vi "log analysis_gps.vi"() -> ()   [LabVIEW 2019] (continued)
#DUALANTENNAHEADINGA,USB3,0,46.5,FINESTEERING,2107,282472.200,02000000,d426,15824;SOL_COMPUTED,L1_FLOAT,-1.000000000,54.732860565,-45.831329346,0.0,98.283119202,178.546401978,\"631T\",13,7,7,7,04,00,20,02*8ccffb99\n\tsystem status\tnormal 2 27.800000 0 0\trobot status\t337.454668\t28.997439\t11.768500\t0.229132\t0.985009\t-32.902606\t0.246000\t0.087000\n\t\n15:27:34.7\tlog_raw\tgps_raw\t#DUALANTENNAHEADINGA,USB3,0,46.5,FINESTEERING,2107,282472.700,02000000,d426,15824;SOL_COMPUTED,L1_FLOAT,-1.000000000,54.959995270,-45.596282959,0.0,98.333869934,179.821563721,\"631T\",13,7,7,7,04,00,20,02*00d3f37b\n\tsystem status\tnormal 2 27.800000 0 0\trobot status\t337.564510\t28.905721\t11.771200\t0.209692\t1.150870\t-32.233289\t0.308000\t-0.003000\n\t\n15:27:35.2\tlog_raw\tgps_raw\t#INSPVAXA,USB3,0,52.0,FINESTEERING,2107,282473.250,02000000,471d,15824;INS_ALIGNMENT_COMPLETE,INS_RTKFIXED,37.37038981275,126.72464739191,11.7746,22.3000,-0.1948,0.2277,0.0045,0.156747113,1.075368694,121.414050270,0.4373,0.2954,0.5425,0.1142,0.0935,0.0768,0.1366,0.1413,5.0978,0f000001,0*e88bca5a\n\tsystem status\tnormal 2 27.700000 0 0\trobot status\t337.686121\t28.806584\t11.774600\t0.156747\t1.075369\t-31.414050\t0.163000\t0.223000\n\t\n15:27:35.7\tlog_raw\tgps_raw\t#INSPVAXA,USB3,0,52.0,FINESTEERING,2107,282473.750,02000000,471d,15824;INS_ALIGNMENT_COMPLETE,INS_RTKFIXED,37.37038901794,126.72464863796,11.7783,22.3000,-0.1909,0.2328,0.0045,0.039175910,1.239409114,120.698239025,0.4373,0.2954,0.5425,0.1142,0.0935,0.0768,0.1366,0.1413,5.0978,0f000001,0*6f6aad10\n\tsystem status\tnormal 2 27.800000 0 0\trobot status\t337.796494\t28.718368\t11.778300\t0.039176\t1.239409\t-30.698239\t0.319000\t0.000000\n\t\n15:27:36.2\tlog_raw\tgps_raw\t#INSPVAXA,USB3,0,52.5,FINESTEERING,2107,282474.250,02000000,471d,15824;INS_ALIGNMENT_COMPLETE,INS_RTKFIXED,37.37038821663,126.72464993203,11.7822,22.3000,-0.1900,0.2213,-0.0032,0.050457416,1.361079347,119.957675424,0.4373,0.2953,0.5423,0.1143,0.0936,0.0767,0.1365,0.1412,5.0971,0f000001,0*04eefe7e\n\tsystem status\tnormal 2 27.800000 0 0\trobot status\t337.911121\t28.629430\t11.782200\t0.050457\t1.361079\t-29.957675\t0.355000\t-0.045000\n\t\n15:27:36.7\tlog_raw\tgps_raw\t#DUALANTENNAHEADINGA,USB3,0,52.5,FINESTEERING,2107,282474.700,02000000,d426,15824;SOL_COMPUTED,NARROW_FLOAT,-1.000000000,53.444328308,-36.252197266,0.0,99.495506287,180.000000000,\"631T\",13,7,7,7,04,00,20,03*a63b34b7\n\tsystem status\tnormal 2 27.800000 0 0\trobot status\t338.015790\t28.551056\t11.786100\t0.032591\t1.365886\t-29.248253\t0.330000\t-0.043000\n\t\n15:27:37.2\tlog_raw\tgps_raw\t\tsystem status\tnormal 2 27.800000 0 0\trobot status\t338.132602\t28.464845\t11.789800\t0.076114\t1.461863\t-28.564426\t0.425000\t-0.155000\n\t\n15:27:37.7\tlog_raw\tgps_raw\t#INSPVAXA,USB3,0,51.0,FINESTEERING,2107,282475.750,02000000,471d,15824;INS_ALIGNMENT_COMPLETE,INS_RTKFIXED,37.37038590363,126.72465390655,11.7950,22.3000,-0.1808,0.2394,-0.0047,0.109913426,1.377387594,117.860298903,0.4381,0.2954,0.5423,0.1145,0.0936,0.0767,0.1364,0.1410,5.0959,0f000001,0*7de89cb0\n\tsystem status\tnormal 2 27.800000 0 0\trobot status\t338.263177\t28.372709\t11.795000\t0.109913\t1.377388\t-27.860299\t0.307000\t-0.004000\n\t\n15:27:38.2\tlog_raw\tgps_raw\t#DUALANTENNAHEADINGA,USB3,0,51.5,FINESTEERING,2107,282476.200,02000000,d426,15824;SOL_COMPUTED,L1_FLOAT,-1.000000000,55.533638000,-0.375610352,0.0,117.860015869,180.000000000,\"631T\",14,7,7,7,04,00,20,02*d327ff6e\n\tsystem status\tnormal 2 27.800000 0 0\trobot status\t338.370911\t28.297956\t11.799000\t0.118267\t1.261755\t-27.251157\t0.371000\t-0.097000\n\t\n15:27:38.7\tlog_raw\tgps_raw\t#INSPVAXA,USB3,0,51.5,FINESTEERING,2107,282476.750,02000000,471d,15824;INS_ALIGNMENT_COMPLETE,INS_RTKFIXED,37.37038443010,126.72465662645,11.8037,22.3000,-0.1744,0.2321,0.0038,0.098053038,1.110033651,116.595542201,0.4382,0.2952,0.5423,0.1147,0.0936,0.0767,0.1363,0.1408,5.0950,0f000001,0*ea8caedb\n\tsystem status\tnormal 2 27.800000 0 0\trobot status\t338.504102\t28.209160\t11.803700\t0.098053\t1.110034\t-26.595542\t0.263000\t0.066000\n\t\n15:27:39.2\tlog_raw\tgps_raw\t#INSPVAXA,USB3,0,52.0,FINESTEERING,2107,282477.250,02000000,471d,15824;INS_ALIGNMENT_COMPLETE,INS_RTKFIXED,37.37038371373,126.72465798496,11.8086,22.3000,-0.1784,0.2376,0.0072,0.132722378,1.123390738,116.043560691,0.4382,0.2951,0.5421,0.1149,0.0937,0.0767,0.1362,0.1405,5.0949,0f000001,0*a21a9ce6\n\tsystem status\tnormal 2 27.800000 0 0\trobot status\t338.624436\t28.129649\t11.808600\t0.132722\t1.123391\t-26.043561\t0.236000\t0.120000\n\t\n15:27:39.7\tlog_raw\tgps_raw\t\tsystem status\tnormal 2 27.800000 0 0\trobot status\t338.734436\t28.057677\t11.812800\t0.158038\t0.982848\t-25.549618\t0.227000\t0.142000\n\t\n15:27:40.2\tlog_raw\tgps_raw\t#DUALANTENNAHEADINGA,USB3,0,47.5,FINESTEERING,2107,282478.200,02000000,d426,15824;SOL_COMPUTED,NARROW_FLOAT,-1.000000000,53.676605225,18.221975327,0.0,112.330833435,180.000000000,\"631T\",17,7,7,7,04,00,20,03*123ff075\n\tsystem status\tnormal 2 27.800000 0 0\trobot status\t338.855171\t27.980159\t11.816500\t0.150261\t1.168449\t-25.066939\t0.205000\t0.163000\n\t\n15:27:40.7\tlog_raw\tgps_raw\t#INSPVAXA,USB3,0,47.5,FINESTEERING,2107,282478.750,02000000,471d,15824;INS_ALIGNMENT_COMPLETE,INS_RTKFIXED,37.37038162641,126.72466209113,11.8198,22.3000,-0.1768,0.2383,-0.0098,0.146556317,1.371576994,114.526516784,0.4387,0.2951,0.5427,0.1151,0.0939,0.0768,0.1361,0.1403,5.0955,0f000001,0*9c50f9d9\n\tsystem status\tnormal 2 27.800000 0 0\trobot status\t338.988154\t27.897974\t11.819800\t0.146556\t1.371577\t-24.526517\t0.228000\t0.129000\n\t\n15:27:41.2\tlog_raw\tgps_raw\t#DUALANTENNAHEADINGA,USB3,0,50.0,FINESTEERING,2107,282479.200,02000000,d426,15824;SOL_COMPUTED,NARROW_FLOAT,-1.000000000,51.679660797,16.235267639,0.0,131.237731934,180.000000000,\"631T\",15,7,7,7,04,00,20,03*76498f9b\n\tsystem status\tnormal 2 27.900000 0 0\trobot status\t339.098405\t27.832776\t11.821900\t-0.028367\t1.309021\t-24.118833\t0.237000\t0.114000\n\t\n15:27:41.7\tlog_raw\tgps_raw\t#INSPVAXA,USB3,0,50.0,FINESTEERING,2107,282479.750,02000000,471d,15824;INS_ALIGNMENT_COMPLETE,INS_RTKFIXED,37.37038033615,126.72466486857,11.8253,22.3000,-0.1778,0.2630,-0.0031,-0.080326690,1.236523677,113.540262033,0.4414,0.2959,0.5454,0.1157,0.0941,0.0769,0.1359,0.1401,5.0966,0f000001,0*bc5588b9\n\tsystem status\tnormal 2 27.900000 0 0\trobot status\t339.234175\t27.754765\t11.825300\t-0.080327\t1.236524\t-23.540262\t0.233000\t0.109000\n\t\n15:27:42.2\tlog_raw\tgps_raw\t\tsystem status\tnormal 2 27.900000 0 0\trobot status\t339.345086\t27.692770\t11.827000\t-0.206343\t1.191786\t-23.092639\t0.254000\t0.074000\n\t\n15:27:42.7\tlog_raw\tgps_raw\t#INSPVAXA,USB3,0,51.0,FINESTEERING,2107,282480.750,02000000,471d,15824;INS_ALIGNMENT_COMPLETE,INS_RTKFIXED,37.37037910395,126.72466763539,11.8294,22.3000,-0.1682,0.2496,-0.0083,-0.123932791,1.123250163,112.586404178,0.4418,0.2960,0.5463,0.1157,0.0942,0.0770,0.1357,0.1398,5.0977,0f000001,0*a24ca24f\n\tsystem status\tnormal 2 27.900000 0 0\trobot status\t339.479256\t27.618000\t11.829400\t-0.123933\t1.123250\t-22.586404\t0.323000\t-0.027000\n\t\n15:27:43.2\tlog_raw\tgps_raw\t\tsystem status\tnormal 2 27.900000 0 0\trobot status\t339.593893\t27.557561\t11.831700\t-0.289570\t1.176785\t-22.187995\t0.299000\t0.006000\n\t\n15:27:43.7\tlog_raw\tgps_raw\t#INSPVAXA,USB3,0,49.5,FINESTEERING,2107,282481.750,02000000,471d,15824;INS_ALIGNMENT_COMPLETE,INS_RTKFIXED,37.37037789694,126.72467048931,11.8351,22.3000,-0.1461,0.2327,0.0043,-0.310804253,1.123961293,111.895191809,0.4415,0.2959,0.5463,0.1157,0.0942,0.0769,0.1355,0.1395,5.0988,0f000001,0*973dff57\n\tsystem status\tnormal 2 27.900000 0 0\trobot status\t339.732051\t27.484030\t11.835100\t-0.310804\t1.123961\t-21.895192\t0.346000\t-0.056000\n\t\n15:27:44.2\tlog_raw\tgps_raw\t#INSPVAXA,USB3,0,50.5,FINESTEERING,2107,282482.250,02000000,471d,15824;INS_ALIGNMENT_COMPLETE,INS_RTKFIXED,37.37037731116,126.72467190347,11.8384,22.3000,-0.1477,0.2523,-0.0105,-0.265666832,1.108878256,111.633485530,0.4404,0.2956,0.5456,0.1156,0.0941,0.0769,0.1353,0.1392,5.0999,0f000001,0*cd6558ee\n\tsystem status\tnormal 2 27.900000 0 0\trobot status\t339.857315\t27.419012\t11.838400\t-0.265667\t1.108878\t-21.633486\t0.243000\t0.085000\n\t\n15:27:44.7\tlog_raw\tgps_raw\t#INSPVAXA,USB3,0,50.5,FINESTEERING,2107,282482.750,02000000,471d,15824;INS_ALIGNMENT_COMPLETE,INS_RTKFIXED,37.37037674280,126.72467330399,11.8420,22.3000,-0.1430,0.2494,-0.0020,-0.174444219,1.137466494,111.346444953,0.4404,0.2956,0.5456,0.1156,0.0941,0.0769,0.1353,0.1392,5.0999,0f000001,0*2a49352f\n\tsystem status\tnormal 2 27.900000 0 0\trobot status\t339.981371\t27.355928\t11.842000\t-0.174444\t1.137466\t-21.346445\t0.276000\t0.036000\n\t\n15:27:45.2\tlog_raw\tgps_raw\t#INSPVAXA,USB3,0,50.0,FINESTEERING,2107,282483.250,02000000,471d,15824;INS_ALIGNMENT_COMPLETE,INS_RTKFIXED,37.37037616883,126.72467474324,11.8449,22.3000,-0.1483,0.2627,-0.0049,-0.159355428,1.028327028,111.093660255,0.4396,0.2956,0.5446,0.1155,0.0941,0.0768,0.1351,0.1389,5.1012,0f000001,0*e9226b16\n\tsystem status\tnormal 2 28.000000 0 0\trobot status\t340.108857\t27.292221\t11.844900\t-0.159355\t1.028327\t-21.093660\t0.334000\t-0.044000\n\t\n15:27:45.7\tlog_raw\tgps_raw\t#INSPVAXA,USB3,0,50.0,FINESTEERING,2107,282483.750,02000000,471d,15824;INS_ALIGNMENT_COMPLETE,INS_RTKFIXED,37.37037559924,126.72467616191,11.8460,22.3000,-0.1456,0.2485,-0.0071,-0.147252002,0.996738159,110.847183596,0.4396,0.2956,0.5446,0.1155,0.0941,0.0768,0.1351,0.1389,5.1012,0f000001,0*6063b49d\n\tsystem status\tnormal 2 28.000000 0 0\trobot status\t340.234521\t27.229000\t11.846000\t-0.147252\t0.996738\t-20.847184\t0.323000\t-0.029000\n\t\n15:27:46.2\tlog_raw\tgps_raw\t\tsystem status\tnormal 2 28.000000 0 0\trobot status\t340.347700\t27.173384\t11.848500\t-0.118940\t0.919299\t-20.556192\t0.292000\t0.033000\n\t\n15:27:46.7\tlog_raw\tgps_raw\t#INSPVAXA,USB3,0,51.5,FINESTEERING,2107,282484.750,02000000,471d,15824;INS_ALIGNMENT_COMPLETE,INS_RTKFIXED,37.37037448665,126.72467902626,11.8522,22.3000,-0.1407,0.2484,-0.0090,-0.064873099,1.145438573,110.168729835,0.4390,0.2955,0.5438,0.1153,0.0940,0.0767,0.1348,0.1386,5.1026,0f000001,0*a0636209\n\tsystem status\tnormal 2 27.900000 0 0\trobot status\t340.488240\t27.105510\t11.852200\t-0.064873\t1.145439\t-20.168730\t0.418000\t-0.152000\n\t\n15:27:47.2\tlog_raw\tgps_raw\t#INSPVAXA,USB3,0,51.0,FINESTEERING,2107,282485.250,02008000,471d,15824;INS_ALIGNMENT_COMPLETE,INS_RTKFIXED,37.37037393424,126.72468050363,11.8549,22.3000,-0.1324,0.2566,-0.0083,0.002695886,0.976355436,109.894464634,0.4390,0.2956,0.5434,0.1153,0.0939,0.0767,0.1346,0.1383,5.1041,0f000001,0*d70e669a\n\tsystem status\tnormal 2 27.900000 0 0\trobot status\t340.619103\t27.044195\t11.854900\t0.002696\t0.976355\t-19.894465\t0.328000\t-0.009000\n\t\n15:27:47.7\tlog_raw\tgps_raw\t#INSPVAXA,USB3,0,51.0,FINESTEERING,2107,282485.750,02008000,471d,15824;INS_ALIGNMENT_COMPLETE,INS_RTKFIXED,37.37037339561,126.72468193841,11.8561,22.3000,-0.1291,0.2465,-0.0040,0.117309078,0.863917654,109.567582429,0.4390,0.2956,0.5434,0.1153,0.0939,0.0767,0.1346,0.1383,5.1041,0f000001,0*167aa476\n\tsystem status\tnormal 2 27.900000 0 0\trobot status\t340.746194\t26.984411\t11.856100\t0.117309\t0.863918\t-19.567582\t0.358000\t-0.067000\n\t\n15:27:48.2\tlog_raw\tgps_raw\t#DUALANTENNAHEADINGA,USB3,0,52.0,FINESTEERING,2107,282486.200,02008000,d426,15824;SOL_COMPUTED,L1_FLOAT,-1.000000000,124.986564636,-52.100769043,0.0,360.000000000,180.000000000,\"631T\",12,6,6,6,04,00,20,02*25d98b4c\n\tsystem status\tnormal 2 27.900000 0 0\trobot status\t340.861761\t26.930390\t11.857200\t0.186163\t0.788623\t-19.301415\t0.403000\t-0.141000\n\t\n15:27:48.7\tlog_raw\tgps_raw\t#INSPVAXA,USB3,0,52.0,FINESTEERING,2107,282486.750,02008000,471d,15824;INS_ALIGNMENT_COMPLETE,INS_RTKFIXED,37.37037231578,126.72468487356,11.8580,22.3000,-0.1363,0.2539,-0.0079,0.065083536,0.658526684,108.961373177,0.4389,0.2956,0.5429,0.1152,0.0940,0.0767,0.1344,0.1380,5.1058,0f000001,0*795b201f\n\tsystem status\tnormal 2 27.900000 0 0\trobot status\t341.006184\t26.864555\t11.858000\t0.065084\t0.658527\t-18.961373\t0.271000\t0.041000\n\t\n15:27:49.2\tlog_raw\tgps_raw\t\tsystem status\tnormal 2 27.900000 0 0\trobot status\t341.122740\t26.810458\t11.859800\t0.109645\t0.579824\t-18.720730\t0.424000\t-0.184000\n\t\n15:27:49.7\tlog_raw\tgps_raw\t#INSPVAXA,USB3,0,53.0,FINESTEERING,2107,282487.750,02008000,471d,15824;INS_ALIGNMENT_COMPLETE,INS_RTKFIXED,37.37037124612,126.72468781330,11.8615,22.3000,-0.1351,0.2529,-0.0014,0.028036761,0.509941288,108.259170524,0.4390,0.2956,0.5427,0.1151,0.0939,0.0767,0.1342,0.1378,5.1072,0f000001,0*7116cc62\n\tsystem status\tnormal 2 27.900000 0 0\trobot status\t341.266582\t26.745829\t11.861500\t0.028037\t0.509941\t-18.259171\t0.398000\t-0.147000\n\t\n15:27:50.2\tlog_raw\tgps_raw\t\tsystem status\tnormal 2 27.900000 0 0\trobot status\t341.382407\t26.694008\t11.863500\t0.059660\t0.738081\t-17.950165\t0.237000\t0.109000\n\t\n15:27:50.7\tlog_raw\tgps_raw\t#INSPVAXA,USB3,0,50.5,FINESTEERING,2107,282488.750,02008000,471d,15824;INS_ALIGNMENT_COMPLETE,INS_RTKFIXED,37.37037023523,126.72469074006,11.8656,22.3000,-0.1204,0.2670,0.0002,0.044873893,0.831014389,107.580535120,0.4389,0.2956,0.5425,0.1150,0.0937,0.0767,0.1339,0.1375,5.1082,0f000001,0*4cab4b69\n\tsystem status\tnormal 2 27.900000 0 0\trobot status\t341.525829\t26.633625\t11.865600\t0.044874\t0.831014\t-17.580535\t0.245000\t0.092000\n\t\n15:27:51.2\tlog_raw\tgps_raw\t#INSPVAXA,USB3,0,51.0,FINESTEERING,2107,282489.250,02000000,471d,15824;INS_ALIGNMENT_COMPLETE,INS_RTKFIXED,37.37036974630,126.72469219938,11.8668,22.3000,-0.1082,0.2562,0.0055,0.037042210,0.796968035,107.199262674,0.4392,0.2956,0.5428,0.1149,0.0936,0.0767,0.1337,0.1373,5.1092,0f000001,0*9fc09916\n\tsystem status\tnormal 2 27.900000 0 0\trobot status\t341.655094\t26.579356\t11.866800\t0.037042\t0.796968\t-17.199263\t0.281000\t0.033000\n\t\n15:27:51.7\tlog_raw\tgps_raw\t\tsystem status\tnormal 2 27.900000 0 0\trobot status\t341.772406\t26.530600\t11.867400\t-0.037262\t1.019759\t-16.874243\t0.281000\t0.031000\n\t\n15:27:52.2\tlog_raw\tgps_raw\t#INSPVAXA,USB3,0,52.0,FINESTEERING,2107,282490.250,02000000,471d,15824;INS_ALIGNMENT_COMPLETE,INS_RTKFIXED,37.37036877450,126.72469515177,11.8697,22.3000,-0.1086,0.2580,0.0081,-0.074758775,1.106093430,106.454761549,0.4393,0.2955,0.5430,0.1148,0.0934,0.0768,0.1335,0.1371,5.1102,0f000001,0*37127645\n\tsystem status\tnormal 2 27.900000 0 0\trobot status\t341.916611\t26.471491\t11.869700\t-0.074759\t1.106093\t-16.454762\t0.203000\t0.151000\n\t\n15:27:52.7\tlog_raw\tgps_raw\t#INSPVAXA,USB3,0,52.0,FINESTEERING,2107,282490.750,02000000,471d,15824;INS_ALIGNMENT_COMPLETE,INS_RTKFIXED,37.37036829389,126.72469663971,11.8737,22.3000,-0.1049,0.2625,0.0062,-0.116881471,1.024892331,106.058307514,0.4393,0.2955,0.5430,0.1148,0.0934,0.0768,0.1335,0.1371,5.1102,0f000001,0*7841381f\n\tsystem status\tnormal 2 27.900000 0 0\trobot status\t342.048411\t26.418145\t11.873700\t-0.116881\t1.024892\t-16.058308\t0.269000\t0.064000\n\t\n15:27:53.2\tlog_raw\tgps_raw\t#INSPVAXA,USB3,0,51.5,FINESTEERING,2107,282491.250,02000000,471d,15824;INS_ALIGNMENT_COMPLETE,INS_RTKFIXED,37.37036783071,126.72469814477,11.8773,22.3000,-0.1005,0.2703,0.0019,-0.302758145,0.967035823,105.571562776,0.4390,0.2953,0.5427,0.1146,0.0933,0.0767,0.1334,0.1370,5.1117,0f000001,0*df8a40e1\n\tsystem status\tnormal 2 28.000000 0 0\trobot status\t342.181726\t26.366734\t11.877300\t-0.302758\t0.967036\t-15.571563\t0.275000\t0.058000\n\t\n15:27:53.7\tlog_raw\tgps_raw\t\tsystem status\tnormal 2 27.900000 0 0\trobot status\t342.301044\t26.320984\t11.881500\t-0.457558\t0.959747\t-15.154789\t0.307000\t0.003000\n\t\n15:27:54.2\tlog_raw\tgps_raw\t#INSPVAXA,USB3,0,53.0,FINESTEERING,2107,282492.250,02000000,471d,15824;INS_ALIGNMENT_COMPLETE,INS_RTKFIXED,37.37036690492,126.72470114805,11.8868,22.3000,-0.1128,0.2686,-0.0005,-0.341749532,1.011987346,104.657671438,0.4386,0.2951,0.5424,0.1145,0.0933,0.0767,0.1332,0.1368,5.1133,0f000001,0*36e30592\n\tsystem status\tnormal 2 27.900000 0 0\trobot status\t342.447752\t26.263974\t11.886800\t-0.341750\t1.011987\t-14.657671\t0.395000\t-0.113000\n\t\n15:27:54.7\tlog_raw\tgps_raw\t#INSPVAXA,USB3,0,53.0,FINESTEERING,2107,282492.750,02000000,471d,15824;INS_ALIGNMENT_COMPLETE,INS_RTKFIXED,37.37036645131,126.72470265161,11.8901,22.3000,-0.1035,0.2695,-0.0047,-0.206753293,0.813426880,104.258109250,0.4386,0.2951,0.5424,0.1145,0.0933,0.0767,0.1332,0.1368,5.1133,0f000001,0*577226f1\n\tsystem status\tnormal 2 27.900000 0 0\trobot status\t342.580935\t26.213625\t11.890100\t-0.206753\t0.813427\t-14.258109\t0.242000\t0.099000\n\t\n15:27:55.2\tlog_raw\tgps_raw\t#INSPVAXA,USB3,0,50.0,FINESTEERING,2107,282493.250,02000000,471d,15824;INS_ALIGNMENT_COMPLETE,INS_RTKFIXED,37.37036601456,126.72470416352,11.8919,22.3000,-0.1012,0.2672,-0.0093,-0.224228213,0.685864648,103.742995644,0.4383,0.2950,0.5422,0.1144,0.0932,0.0767,0.1331,0.1366,5.1149,0f000001,0*31397ff1\n\tsystem status\tnormal 2 27.800000 0 0\trobot status\t342.714857\t26.165147\t11.891900\t-0.224228\t0.685865\t-13.742996\t0.219000\t0.126000\n\t\n15:27:55.7\tlog_raw\tgps_raw\t#INSPVAXA,USB3,0,50.0,FINESTEERING,2107,282493.750,02000000,471d,15824;INS_ALIGNMENT_COMPLETE,INS_RTKFIXED,37.37036559899,126.72470566002,11.8945,22.3000,-0.1067,0.2704,-0.0029,-0.332770610,0.803747172,103.266979310,0.4383,0.2950,0.5422,0.1144,0.0932,0.0767,0.1331,0.1366,5.1149,0f000001,0*9ccbb3e3\n\tsystem status\tnormal 2 27.800000 0 0\trobot status\t342.847415\t26.119020\t11.894500\t-0.332771\t0.803747\t-13.266979\t0.254000\t0.083000\n\t\n15:27:56.2\tlog_raw\tgps_raw\t#INSPVAXA,USB3,0,54.0,FINESTEERING,2107,282494.250,02000000,471d,15824;INS_ALIGNMENT_COMPLETE,INS_RTKFIXED,37.37036518833,126.72470716061,11.8982,22.3000,-0.0992,0.2825,-0.0009,-0.390155029,0.844314939,102.750620694,0.4383,0.2950,0.5423,0.1144,0.0933,0.0767,0.1329,0.1365,5.1164,0f000001,0*37164162\n\tsystem status\tnormal 2 27.900000 0 0\trobot status\t342.980335\t26.073438\t11.898200\t-0.390155\t0.844315\t-12.750621\t0.238000\t0.095000\n\t\n15:27:56.7\tlog_raw\tgps_raw\t#INSPVAXA,USB3,0,54.0,FINESTEERING,2107,282494.750,02000000,471d,15824;INS_ALIGNMENT_COMPLETE,INS_RTKFIXED,37.37036477713,126.72470868073,11.9009,22.3000,-0.0879,0.2706,0.0036,-0.341565952,0.784824904,102.134248180,0.4383,0.2950,0.5423,0.1144,0.0933,0.0767,0.1329,0.1365,5.1164,0f000001,0*6a9baff3\n\tsystem status\tnormal 2 27.800000 0 0\trobot status\t343.114985\t26.027795\t11.900900\t-0.341566\t0.784825\t-12.134248\t0.294000\t0.017000\n\t\n15:27:57.2\tlog_raw\tgps_raw\t\tsystem status\tnormal 2 27.800000 0 0\trobot status\t343.237786\t25.988898\t11.902700\t-0.374669\t0.912618\t-11.541175\t0.272000\t0.062000\n\t\n15:27:57.7\tlog_raw\tgps_raw\t#INSPVAXA,USB3,0,52.0,FINESTEERING,2107,282495.750,02000000,471d,15824;INS_ALIGNMENT_COMPLETE,INS_RTKFIXED,37.37036401120,126.72471176105,11.9046,22.3000,-0.0834,0.2786,-0.0076,-0.308157155,0.761064852,100.941117040,0.4380,0.2949,0.5422,0.1143,0.0933,0.0767,0.1328,0.1363,5.1178,0f000001,0*054ad5c7\n\tsystem status\tnormal 2 27.800000 0 0\trobot status\t343.387834\t25.942777\t11.904600\t-0.308157\t0.761065\t-10.941117\t0.298000\t0.027000\n\t\n15:27:58.2\tlog_raw\tgps_raw\t#INSPVAXA,USB3,0,50.5,FINESTEERING,2107,282496.250,02000000,471d,15824;INS_ALIGNMENT_COMPLETE,INS_RTKFIXED,37.37036364901,126.72471328274,11.9089,22.3000,-0.0739,0.2539,-0.0014,-0.343894984,0.754370105,100.232900120,0.4379,0.2949,0.5421,0.1143,0.0933,0.0767,0.1327,0.1362,5.1190,0f000001,0*8784bafb\n\tsystem status\tnormal 2 27.800000 0 0\trobot status\t343.522623\t25.902574\t11.908900\t-0.343895\t0.754370\t-10.232900\t0.196000\t0.177000\n\t\n15:27:58.7\tlog_raw\tgps_raw\t#INSPVAXA,USB3,0,50.5,FINESTEERING,2107,282496.750,02000000,471d,15824;INS_ALIGNMENT_COMPLETE,INS_RTKFIXED,37.37036328787,126.72471481476,11.9136,22.3000,-0.0700,0.2693,-0.0009,-0.270371003,0.729660939,99.468887752,0.4379,0.2949,0.5421,0.1143,0.0933,0.0767,0.1327,0.1362,5.1190,0f000001,0*224a36a2\n\tsystem status\tnormal 2 27.800000 0 0\trobot status\t343.658327\t25.862488\t11.913600\t-0.270371\t0.729661\t-9.468888\t0.272000\t0.081000\n\t\n15:27:59.2\tlog_raw\tgps_raw\t#INSPVAXA,USB3,0,52.0,FINESTEERING,2107,282497.250,02000000,471d,15824;INS_ALIGNMENT_COMPLETE,INS_RTKFIXED,37.37036295953,126.72471635660,11.9170,22.3000,-0.0692,0.2638,0.0039,-0.487791758,0.697577068,98.688104249,0.4380,0.2950,0.5422,0.1144,0.0934,0.0767,0.1326,0.1361,5.1201,0f000001,0*5983bd1e\n\tsystem status\tnormal 2 27.800000 0 0\trobot status\t343.794901\t25.826042\t11.917000\t-0.487792\t0.697577\t-8.688104\t0.232000\t0.118000\n\t\n15:27:59.7\tlog_raw\tgps_raw\t#INSPVAXA,USB3,0,52.0,FINESTEERING,2107,282497.750,02000000,471d,15824;INS_ALIGNMENT_COMPLETE,INS_RTKFIXED,37.37036264142,126.72471787968,11.9197,22.3000,-0.0695,0.2760,-0.0054,-0.578412192,0.764831938,97.837503717,0.4380,0.2950,0.5422,0.1144,0.0934,0.0767,0.1326,0.1361,5.1201,0f000001,0*bf0827fb\n\tsystem status\tnormal 2 27.700000 0 0\trobot status\t343.929812\t25.790731\t11.919700\t-0.578412\t0.764832\t-7.837504\t0.312000\t0.003000\n\t\n15:28:00.2\tlog_raw\tgps_raw\t#INSPVAXA,USB3,0,50.5,FINESTEERING,2107,282498.250,02000000,471d,15824;INS_ALIGNMENT_COMPLETE,INS_RTKFIXED,37.37036233909,126.72471942444,11.9220,22.3000,-0.0554,0.2842,0.0042,-0.538460345,0.850776558,96.860804388,0.4376,0.2949,0.5421,0.1145,0.0934,0.0767,0.1325,0.1359,5.1211,0f000001,0*e69b7700\n\tsystem status\tnormal 2 27.700000 0 0\trobot status\t344.066645\t25.757171\t11.922000\t-0.538460\t0.850777\t-6.860804\t0.217000\t0.149000\n\t\n15:28:00.7\tlog_raw\tgps_raw\t#INSPVAXA,USB3,0,50.5,FINESTEERING,2107,282498.750,02000000,471d,15824;INS_ALIGNMENT_COMPLETE,INS_RTKFIXED,37.37036207253,126.72472096393,11.9246,22.3000,-0.0513,0.2714,0.0039,-0.548055416,0.760878793,95.595246784,0.4376,0.2949,0.5421,0.1145,0.0934,0.0767,0.1325,0.1359,5.1211,0f000001,0*75d334ae\n\tsystem status\tnormal 2 27.700000 0 0\trobot status\t344.203010\t25.727581\t11.924600\t-0.548055\t0.760879\t-5.595247\t0.291000\t0.035000\n\t\n15:28:01.2\tlog_raw\tgps_raw\t#INSPVAXA,USB3,0,51.0,FINESTEERING,2107,282499.250,02000000,471d,15824;INS_ALIGNMENT_COMPLETE,INS_RTKFIXED,37.37036182665,126.72472251722,11.9274,22.3000,-0.0518,0.2707,0.0042,-0.612176508,0.765223252,94.525809257,0.4377,0.2950,0.5421,0.1146,0.0936,0.0767,0.1324,0.1357,5.1220,0f000001,0*ec8d0c0f\n\tsystem status\tnormal 2 27.600000 0 0\trobot status\t344.340598\t25.700287\t11.927400\t-0.612177\t0.765223\t-4.525809\t0.294000\t0.038000\n\t\n15:28:01.7\tlog_raw\tgps_raw\t#INSPVAXA,USB3,0,51.0,FINESTEERING,2107,282499.750,02000000,471d,15824;INS_ALIGNMENT_COMPLETE,INS_RTKFIXED,37.37036160600,126.72472408768,11.9291,22.3000,-0.0494,0.2821,-0.0083,-0.781502529,0.706412197,93.339152024,0.4377,0.2950,0.5421,0.1146,0.0936,0.0767,0.1324,0.1357,5.1220,0f000001,0*d9b69855\n\tsystem status\tnormal 2 27.700000 0 0\trobot status\t344.479707\t25.675792\t11.929100\t-0.781503\t0.706412\t-3.339152\t0.303000\t0.039000\n\t\n15:28:02.2\tlog_raw\tgps_raw\t#INSPVAXA,USB3,0,53.0,FINESTEERING,2107,282500.250,02000000,471d,15824;INS_ALIGNMENT_COMPLETE,INS_RTKFIXED,37.37036138755,126.72472565119,11.9317,22.3000,-0.0342,0.2702,0.0095,-0.593682831,0.623847561,91.416153722,0.4373,0.2951,0.5419,0.1148,0.0938,0.0767,0.1322,0.1355,5.1229,0f000001,0*07814bab\n\tsystem status\tnormal 2 27.400000 0 0\trobot status\t344.618200\t25.651542\t11.931700\t-0.593683\t0.623848\t-1.416154\t0.290000\t0.144000\n\t\n15:28:02.7\tlog_raw\tgps_raw\t#INSPVAXA,USB3,0,53.0,FINESTEERING,2107,282500.750,02000000,471d,15824;INS_ALIGNMENT_COMPLETE,INS_RTKFIXED,37.37036130198,126.72472720567,11.9351,22.3000,0.0292,0.2886,0.0019,-0.781993907,0.527535072,86.351201750,0.4373,0.2951,0.5419,0.1148,0.0938,0.0767,0.1322,0.1355,5.1229,0f000001,0*6a6ac25a\n\tsystem status\tnormal 2 27.200000 0 0\trobot status\t344.755893\t25.642039\t11.935100\t-0.781994\t0.527535\t3.648798\t0.283000\t0.183000\n\t\n15:28:03.2\tlog_raw\tgps_raw\t#INSPVAXA,USB3,0,50.5,FINESTEERING,2107,282501.250,02000000,471d,15824;INS_ALIGNMENT_COMPLETE,INS_RTKFIXED,37.37036131745,126.72472879768,11.9390,22.3000,0.0369,0.2857,-0.0120,-0.997390809,0.433664742,81.039166738,0.4370,0.2954,0.5418,0.1155,0.0947,0.0767,0.1321,0.1353,5.1226,0f000001,0*2c9768ec\n\tsystem status\tnormal 2 27.100000 4 0\trobot status\t344.896911\t25.643751\t11.939000\t-0.997391\t0.433665\t8.960833\t0.311000\t0.166000\n\t\n15:28:03.7\tlog_raw\tgps_raw\t#INSPVAXA,USB3,0,50.5,FINESTEERING,2107,282501.750,02000000,471d,15824;INS_ALIGNMENT_COMPLETE,INS_RTKFIXED,37.37036141879,126.72473040754,11.9428,22.3000,0.0024,0.2788,-0.0052,-1.183204075,0.224327122,76.081887809,0.4370,0.2954,0.5418,0.1155,0.0947,0.0767,0.1321,0.1353,5.1226,0f000001,0*e82bc0a6\n\tsystem status\tnormal 2 27.300000 4 0\trobot status\t345.039510\t25.654992\t11.942800\t-1.183204\t0.224327\t13.918112\t0.325000\t0.168000\n\t\n15:28:04.2\tlog_raw\tgps_raw\t#INSPVAXA,USB3,0,52.5,FINESTEERING,2107,282502.250,02000000,471d,15824;INS_ALIGNMENT_COMPLETE,INS_RTKFIXED,37.37036164481,126.72473194519,11.9462,22.3000,0.0415,0.2803,0.0079,-1.160166771,-0.046948160,70.699699998,0.4369,0.2959,0.5417,0.1169,0.0967,0.0767,0.1320,0.1349,5.1194,0f000001,0*06dae310\n\tsystem status\tnormal 2 27.200000 4 0\trobot status\t345.175712\t25.680071\t11.946200\t-1.160167\t-0.046948\t19.300300\t0.313000\t0.172000\n\t\n15:28:04.7\tlog_raw\tgps_raw\t#INSPVAXA,USB3,0,52.5,FINESTEERING,2107,282502.750,02000000,471d,15824;INS_ALIGNMENT_COMPLETE,INS_RTKFIXED,37.37036200144,126.72473343849,11.9497,22.3000,0.0229,0.2449,0.0184,-1.242261291,-0.215624383,65.570089717,0.4369,0.2959,0.5417,0.1169,0.0967,0.0767,0.1320,0.1349,5.1194,0f000001,0*37a9ba1d\n\tsystem status\tnormal 2 27.100000 4 0\trobot status\t345.307986\t25.719646\t11.949700\t-1.242261\t-0.215624\t24.429910\t0.318000\t0.242000\n\t\n15:28:05.2\tlog_raw\tgps_raw\t#INSPVAXA,USB3,0,50.0,FINESTEERING,2107,282503.250,02000000,471d,15824;INS_ALIGNMENT_COMPLETE,INS_RTKFIXED,37.37036244144,126.72473485715,11.9546,22.3000,0.1159,0.2427,0.0087,-1.370274877,-0.522424319,60.146587364,0.4368,0.2966,0.5416,0.1192,0.0988,0.0767,0.1318,0.1345,5.1111,0f000001,0*9f9b3eba\n\tsystem status\tnormal 2 27.200000 4 0\trobot status\t345.433649\t25.768474\t11.954600\t-1.370275\t-0.522424\t29.853413\t0.306000\t0.172000\n\t\n15:28:05.7\tlog_raw\tgps_raw\t#INSPVAXA,USB3,0,50.0,FINESTEERING,2107,282503.750,02000000,471d,15824;INS_ALIGNMENT_COMPLETE,INS_RTKFIXED,37.37036302784,126.72473625079,11.9579,22.3000,0.1573,0.2456,0.0068,-1.326431987,-0.638529875,54.895159113,0.4368,0.2966,0.5416,0.1192,0.0988,0.0767,0.1318,0.1345,5.1111,0f000001,0*c3a1e695\n\tsystem status\tnormal 2 27.300000 4 0\trobot status\t345.557095\t25.833550\t11.957900\t-1.326432\t-0.638530\t35.104841\t0.298000\t0.165000\n\t\n15:28:06.2\tlog_raw\tgps_raw\t#INSPVAXA,USB3,0,51.0,FINESTEERING,2107,282504.250,02000000,471d,15824;INS_ALIGNMENT_COMPLETE,INS_RTKFIXED,37.37036369327,126.72473758611,11.9611,22.3000,0.1628,0.2237,0.0021,-1.236535008,-0.784458797,49.797084734,0.4377,0.2981,0.5419,0.1224,0.1023,0.0767,0.1314,0.1337,5.1002,0f000001,0*ce2dc0c6\n\tsystem status\tnormal 2 27.200000 4 0\trobot status\t345.675376\t25.907398\t11.961100\t-1.236535\t-0.784459\t40.202915\t0.310000\t0.175000\n\t\n15:28:06.7\tlog_raw\tgps_raw\t#INSPVAXA,USB3,0,51.0,FINESTEERING,2107,282504.750,02000000,471d,15824;INS_ALIGNMENT_COMPLETE,INS_RTKFIXED,37.37036443928,126.72473881419,11.9655,22.3000,0.1771,0.2224,-0.0093,-1.091153284,-0.604631231,44.754867869,0.4377,0.2981,0.5419,0.1224,0.1023,0.0767,0.1314,0.1337,5.1002,0f000001,0*68fd2785\n\tsystem status\tnormal 2 27.200000 4 0\trobot status\t345.784157\t25.990189\t11.965500\t-1.091153\t-0.604631\t45.245132\t0.332000\t0.139000\n\t\n15:28:07.2\tlog_raw\tgps_raw\t#INSPVAXA,USB3,0,51.0,FINESTEERING,2107,282505.250,02000000,471d,15824;INS_ALIGNMENT_COMPLETE,INS_RTKFIXED,37.37036527959,126.72473995022,11.9707,22.3000,0.1963,0.1952,-0.0121,-1.138350697,-0.474117376,39.571733238,0.4394,0.3003,0.5422,0.1267,0.1058,0.0767,0.1307,0.1325,5.0879,0f000001,0*6827ef91\n\tsystem status\tnormal 2 27.100000 4 0\trobot status\t345.884785\t26.083446\t11.970700\t-1.138351\t-0.474117\t50.428267\t0.287000\t0.194000\n\t\n15:28:07.7\tlog_raw\tgps_raw\t#INSPVAXA,USB3,0,51.0,FINESTEERING,2107,282505.750,02000000,471d,15824;INS_ALIGNMENT_COMPLETE,INS_RTKFIXED,37.37036623616,126.72474098646,11.9763,22.3000,0.2120,0.1861,0.0048,-1.165263195,-0.362025094,34.418588384,0.4394,0.3003,0.5422,0.1267,0.1058,0.0767,0.1307,0.1325,5.0879,0f000001,0*40d9afbc\n\tsystem status\tnormal 2 27.200000 4 0\trobot status\t345.976573\t26.189607\t11.976300\t-1.165263\t-0.362025\t55.581412\t0.326000\t0.171000\n\t\n15:28:08.2\tlog_raw\tgps_raw\t#INSPVAXA,USB3,0,51.5,FINESTEERING,2107,282506.250,02000000,471d,15824;INS_ALIGNMENT_COMPLETE,INS_RTKFIXED,37.37036720685,126.72474192456,11.9800,22.3000,0.2212,0.1614,0.0108,-1.132985321,-0.180413000,28.958926810,0.4417,0.3033,0.5424,0.1317,0.1100,0.0768,0.1296,0.1309,5.0779,0f000001,0*2e0d677d\n\tsystem status\tnormal 2 27.200000 4 0\trobot status\t346.059669\t26.297335\t11.980000\t-1.132985\t-0.180413\t61.041073\t0.302000\t0.181000\n\t\n15:28:08.7\tlog_raw\tgps_raw\t#INSPVAXA,USB3,0,51.5,FINESTEERING,2107,282506.750,02000000,471d,15824;INS_ALIGNMENT_COMPLETE,INS_RTKFIXED,37.37036827241,126.72474279747,11.9819,22.3000,0.2642,0.1305,0.0010,-1.072910910,-0.236865707,23.702771649,0.4417,0.3033,0.5424,0.1317,0.1100,0.0768,0.1296,0.1309,5.0779,0f000001,0*c0c775a0\n\tsystem status\tnormal 2 27.100000 4 0\trobot status\t346.136989\t26.415593\t11.981900\t-1.072911\t-0.236866\t66.297228\t0.282000\t0.216000\n\t\n15:28:09.2\tlog_raw\tgps_raw\t#INSPVAXA,USB3,0,51.0,FINESTEERING,2107,282507.250,02000000,471d,15824;INS_ALIGNMENT_COMPLETE,INS_RTKFIXED,37.37036943623,126.72474351475,11.9844,22.3000,0.2890,0.1143,0.0134,-1.116078326,-0.545577808,18.460028821,0.4448,0.3070,0.5424,0.1371,0.1144,0.0767,0.1279,0.1286,5.0714,0f000001,0*f2488cfe\n\tsystem status\tnormal 2 27.000000 4 0\trobot status\t346.200525\t26.544756\t11.984400\t-1.116078\t-0.545578\t71.539971\t0.318000\t0.148000\n\t\n15:28:09.7\tlog_raw\tgps_raw\t\tsystem status\texception 2 27.700000 4 160\trobot status\t346.243737\t26.612990\t11.986800\t-0.886764\t-0.668691\t73.434057\t0.120000\t-0.067000\n\t\n15:28:10.2\tlog_raw\tgps_raw\t#INSPVAXA,USB3,0,49.5,FINESTEERING,2107,282508.250,02000000,471d,15824;INS_ALIGNMENT_COMPLETE,INS_RTKFIXED,37.37036997810,126.72474418441,11.9888,22.3000,-0.0010,0.0343,0.0051,-0.948239100,-0.592787875,16.930139244,0.4486,0.3110,0.5423,0.1420,0.1207,0.0767,0.1255,0.1258,5.0683,0f000001,0*51dd059e\n\tsystem status\texception 2 28.000000 0 160\trobot status\t346.259842\t26.604893\t11.988800\t-0.948239\t-0.592788\t73.069861\t0.103000\t0.156000\n\t\n15:28:10.7\tlog_raw\tgps_raw\t#INSPVAXA,USB3,0,49.5,FINESTEERING,2107,282508.750,02000000,471d,15824;INS_ALIGNMENT_COMPLETE,INS_RTKFIXED,37.37036994386,126.72474436952,11.9909,22.3000,0.0056,0.0342,0.0053,-0.946500303,-0.592283051,16.912290627,0.4486,0.3110,0.5423,0.1420,0.1207,0.0767,0.1255,0.1258,5.0683,0f000001,0*09452605\n\tsystem status\texception 2 28.000000 0 160\trobot status\t346.276239\t26.601092\t11.990900\t-0.946500\t-0.592283\t73.087709\t0.103000\t0.156000\n\t\n15:28:11.2\tlog_raw\tgps_raw\t#INSPVAXA,USB3,0,51.0,FINESTEERING,2107,282509.250,02000000,471d,15824;INS_ALIGNMENT_COMPLETE,INS_RTKFIXED,37.37036993090,126.72474452786,11.9926,22.3000,0.0102,0.0361,0.0058,-0.944896447,-0.590729782,16.915447262,0.4529,0.3176,0.5421,0.1446,0.1223,0.0767,0.1224,0.1224,5.0667,0f000001,0*6e2fa647\n\tsystem status\texception 2 28.000000 0 160\trobot status\t346.290265\t26.599653\t11.992600\t-0.944896\t-0.590730\t73.084553\t0.103000\t0.156000\n\t\n15:28:11.7\tlog_raw\tgps_raw\t\tsystem status\texception 2 28.000000 0 160\trobot status\t346.301631\t26.601055\t11.993800\t-0.944236\t-0.592815\t73.083852\t0.103000\t0.156000\n\t\n15:28:12.2\tlog_raw\tgps_raw\t#INSPVAXA,USB3,0,53.0,FINESTEERING,2107,282510.250,02000000,471d,15824;INS_ALIGNMENT_COMPLETE,INS_RTKFIXED,37.37036996579,126.72474474686,11.9940,22.3000,0.0173,0.0357,0.0059,-0.945727300,-0.590701581,16.921367979,0.4568,0.3226,0.5419,0.1454,0.1213,0.0767,0.1190,0.1189,5.0583,0f000001,0*ffef94ef\n\tsystem status\texception 2 28.000000 0 160\trobot status\t346.309663\t26.603525\t11.994000\t-0.945727\t-0.590702\t73.078632\t0.103000\t0.156000\n\t\n15:28:12.7\tlog_raw\tgps_raw\t\tsystem status\texception 2 28.000000 0 160\trobot status\t346.313655\t26.606935\t11.993200\t-0.945766\t-0.586317\t73.066857\t0.103000\t0.156000\n\t\n15:28:13.2\tlog_raw\tgps_raw\t#INSPVAXA,USB3,0,52.5,FINESTEERING,2107,282511.250,02000000,471d,15824;INS_ALIGNMENT_COMPLETE,INS_RTKFIXED,37.37037004020,126.72474481545,11.9932,22.3000,0.0243,0.0321,0.0064,-0.946167296,-0.585921759,16.948767668,0.4597,0.3251,0.5417,0.1447,0.1186,0.0767,0.1156,0.1154,5.0445,0f000001,0*7b6abdb9\n\tsystem status\texception 2 28.000000 0 160\trobot status\t346.315739\t26.611783\t11.993200\t-0.946167\t-0.585922\t73.051232\t0.103000\t0.156000\n\t\n15:28:13.7\tlog_raw\tgps_raw\t#INSPVAXA,USB3,0,52.5,FINESTEERING,2107,282511.750,02000000,471d,15824;INS_ALIGNMENT_COMPLETE,INS_RTKFIXED,37.37037009329,126.72474481876,11.9942,22.3000,0.0266,0.0296,0.0059,-0.946113144,-0.582976087,16.966624089,0.4597,0.3251,0.5417,0.1447,0.1186,0.0767,0.1156,0.1154,5.0445,0f000001,0*617dc724\n\tsystem status\texception 2 28.000000 0 160\trobot status\t346.316032\t26.617675\t11.994200\t-0.946113\t-0.582976\t73.033376\t0.103000\t0.156000\n\t\n15:28:14.2\tlog_raw\tgps_raw\t#INSPVAXA,USB3,0,52.5,FINESTEERING,2107,282512.250,02000000,471d,15824;INS_ALIGNMENT_COMPLETE,INS_RTKFIXED,37.37037014737,126.72474480897,11.9952,22.3000,0.0300,0.0277,0.0058,-0.945767980,-0.581738683,16.984774160,0.4614,0.3254,0.5416,0.1426,0.1149,0.0767,0.1126,0.1124,5.0293,0f000001,0*18dcd093\n\tsystem status\texception 2 28.000000 0 160\trobot status\t346.315165\t26.623677\t11.995200\t-0.945768\t-0.581739\t73.015226\t0.103000\t0.156000\n\t\n15:28:14.7\tlog_raw\tgps_raw\t\tsystem status\texception 2 28.000000 0 160\trobot status\t346.313390\t26.629735\t11.996300\t-0.945482\t-0.578421\t72.995394\t0.103000\t0.156000\n\t\n15:28:15.2\tlog_raw\tgps_raw\t\tsystem status\texception 2 28.000000 0 160\trobot status\t346.310905\t26.635102\t11.997100\t-0.945925\t-0.578644\t72.975991\t0.103000\t0.156000\n\t\n15:28:15.7\tlog_raw\tgps_raw\t\tsystem status\texception 2 28.000000 0 160\trobot status\t346.307772\t26.639995\t11.997900\t-0.946669\t-0.578776\t72.958003\t0.103000\t0.156000\n\t\n15:28:16.2\tlog_raw\tgps_raw\t\tsystem status\texception 2 28.000000 0 160\trobot status\t346.304326\t26.644527\t11.998300\t-0.945581\t-0.576866\t72.939859\t0.103000\t0.156000\n\t\n15:28:16.7\tlog_raw\tgps_raw\t#INSPVAXA,USB3,0,50.5,FINESTEERING,2107,282514.750,02000000,471d,15824;INS_ALIGNMENT_COMPLETE,INS_RTKFIXED,37.37037037038,126.72474464474,11.9984,22.3000,0.0379,0.0170,0.0059,-0.942581332,-0.576970868,17.074319764,0.4609,0.3217,0.5415,0.1361,0.1072,0.0767,0.1082,0.1079,5.0056,0f000001,0*ba3ae658\n\tsystem status\tnormal 2 28.000000 0 128\trobot status\t346.300618\t26.648428\t11.998400\t-0.942581\t-0.576971\t72.925680\t0.103000\t0.156000\n\t\n15:28:17.2\tlog_raw\tgps_raw\t\tsystem status\texception 2 28.000000 0 160\trobot status\t346.290345\t26.628068\t11.993600\t-0.942987\t-0.571430\t72.894116\t0.103000\t0.156000\n\t\n15:28:17.7\tlog_raw\tgps_raw\t\tsystem status\texception 2 28.000000 0 160\trobot status\t346.273018\t26.580327\t11.983300\t-0.941831\t-0.563461\t72.849649\t0.103000\t0.156000\n\t\n15:28:18.2\tlog_raw\tgps_raw\t\tsystem status\texception 2 28.000000 0 160\trobot status\t346.262825\t26.553588\t11.976800\t-0.937972\t-0.558719\t72.823969\t0.103000\t0.156000\n\t\n15:28:18.7\tlog_raw\tgps_raw\t\tsystem status\texception 2 28.000000 0 160\trobot status\t346.261105\t26.552020\t11.974800\t-0.937823\t-0.559712\t72.821506\t0.103000\t0.156000\n\t\n15:28:19.2\tlog_raw\tgps_raw\t\tsystem status\texception 2 28.000000 0 160\trobot status\t346.259898\t26.551608\t11.973300\t-0.938102\t-0.556302\t72.818046\t0.103000\t0.156000\n\t\n15:28:19.7\tlog_raw\tgps_raw\t\tsystem status\texception 2 28.000000 0 160\trobot status\t346.259531\t26.552747\t11.972600\t-0.937679\t-0.556937\t72.814956\t0.103000\t0.156000\n\t\n15:28:20.2\tlog_raw\tgps_raw\t\tsystem status\texception 2 28.000000 0 160\trobot status\t346.259374\t26.554051\t11.972100\t-0.935936\t-0.559010\t72.811326\t0.103000\t0.156000\n\t\n15:28:20.7\tlog_raw\tgps_raw\t\tsystem status\texception 2 28.000000 0 160\trobot status\t346.259279\t26.555610\t11.971600\t-0.937704\t-0.558863\t72.807878\t0.103000\t0.156000\n\t\n15:28:21.2\tlog_raw\tgps_raw\t\tsystem status\texception 2 28.000000 0 160\trobot status\t346.259020\t26.557032\t11.971300\t-0.936545\t-0.556984\t72.799546\t0.103000\t0.156000\n\t\n15:28:21.7\tlog_raw\tgps_raw\t\tsystem status\texception 2 28.000000 0 160\trobot status\t346.258567\t26.558555\t11.971000\t-0.936467\t-0.554691\t72.789832\t0.103000\t0.156000\n\t\n15:28:22.2\tlog_raw\tgps_raw\t\tsystem status\texception 2 28.000000 0 160\trobot status\t346.258327\t26.560104\t11.970700\t-0.935578\t-0.555207\t72.784559\t0.103000\t0.156000\n\t\n15:28:22.7\tlog_raw\tgps_raw\t\tsystem status\texception 2 28.000000 0 160\trobot status\t346.258432\t26.561408\t11.970300\t-0.933823\t-0.554873\t72.778038\t0.103000\t0.156000\n\t\n15:28:23.2\tlog_raw\tgps_raw\t\tsystem status\texception 2 28.000000 0 160\trobot status\t346.258415\t26.562837\t11.970200\t-0.933538\t-0.552700\t72.772730\t0.103000\t0.156000\n\t\n15:28:23.7\tlog_raw\tgps_raw\t\tsystem status\texception 2 28.000000 0 160\trobot status\t346.258389\t26.564414\t11.970200\t-0.933870\t-0.553827\t72.769106\t0.103000\t0.156000\n\t\n15:28:24.2\tlog_raw\tgps_raw\t\tsystem status\texception 2 28.000000 0 160\trobot status\t346.258404\t26.565975\t11.970200\t-0.934357\t-0.550925\t72.762300\t0.103000\t0.156000\n\t\n15:28:24.7\tlog_raw\tgps_raw\t\tsystem status\texception 2 28.000000 0 160\trobot status\t346.258794\t26.567644\t11.970400\t-0.934655\t-0.550721\t72.758327\t0.103000\t0.156000\n\t\n15:28:25.2\tlog_raw\tgps_raw\t\tsystem status\texception 0 28.000000 0 32\trobot status\t346.259069\t26.568887\t11.970800\t-0.935495\t-0.550894\t72.755995\t0.103000\t0.156000\n\t\n15:28:25.7\tlog_raw\tgps_raw\t\tsystem status\texception 0 28.000000 0 32\trobot status\t346.258727\t26.569400\t11.971000\t-0.935282\t-0.549651\t72.750637\t0.103000\t0.156000\n\t\n15:28:26.3\tlog_raw\tgps_raw\t\tsystem status\texception 0 28.000000 0 32\trobot status\t346.258445\t26.570268\t11.971300\t-0.937622\t-0.548176\t72.742639\t0.103000\t0.156000\n\t\n15:28:26.8\tlog_raw\tgps_raw\t\tsystem status\texception 0 28.000000 0 32\trobot status\t346.258058\t26.571729\t11.971400\t-0.938804\t-0.546458\t72.738301\t0.103000\t0.156000\n\t\n15:28:27.3\tlog_raw\tgps_raw\t\tsystem status\texception 0 28.000000 0 32\trobot status\t346.257651\t26.573064\t11.971700\t-0.938341\t-0.545860\t72.733717\t0.103000\t0.156000\n\t\n15:28:27.8\tlog_raw\tgps_raw\t\tsystem status\texception 0 28.000000 0 32\trobot status\t346.257456\t26.574078\t11.971600\t-0.936822\t-0.543059\t72.729948\t0.103000\t0.156000\n\t\n15:28:28.3\tlog_raw\tgps_raw\t\tsystem status\texception 0 28.000000 0 32\trobot status\t346.257049\t26.574841\t11.971400\t-0.935693\t-0.543788\t72.722894\t0.103000\t0.155000\n\t\n15:28:28.8\tlog_raw\tgps_raw\t\tsystem status\texception 0 28.000000 0 32\trobot status\t346.256441\t26.574823\t11.971400\t-0.937501\t-0.539932\t72.715902\t0.106000\t0.147000\n\t\n15:28:29.3\tlog_raw\tgps_raw\t\tsystem status\texception 0 28.100000 0 60\trobot status\t346.256776\t26.576333\t11.971100\t-0.939953\t-0.546505\t72.595248\t0.097000\t0.019000\n\t\n15:28:29.8\tlog_raw\tgps_raw\t\tsystem status\texception 0 28.100000 0 60\trobot status\t346.257778\t26.580242\t11.970500\t-0.940612\t-0.543792\t72.587058\t0.097000\t0.019000\n\t\n15:28:30.3\tlog_raw\tgps_raw\t\tsystem status\texception 0 28.100000 0 60\trobot status\t346.258654\t26.584645\t
